vi "Exp05_JointAngle.vi"() -> ()   [LabVIEW 2019]
uses:
  <vilib>/myRIO/Instrument Drivers/Onboard IO/I2C/typedefs/I2C User Configuration.ctl
  <vilib>/myRIO/Instrument Drivers/Onboard IO/I2C/typedefs/I2C Transfer Rate.ctl
  <vilib>/Platform/TimedLoop/XDataNode/timing_clust.ctl
  <vilib>/Platform/TimedLoop/XDataNode/nitl_modes.ctl
  <vilib>/Platform/TimedLoop/XDataNode/wakeup.ctl
  <vilib>/Utility/error.llb/Error Cluster From Error Code.vi
  <vilib>/myRIO/Common/Instrument Driver Framework/myRIO v1.0/I2C/vis/myRIO v1.0 Configure I2C.vi
  <vilib>/myRIO/Common/Instrument Driver Framework/myRIO v1.0/I2C/vis/myRIO v1.0 Write I2C.vi
  <vilib>/myRIO/Common/Instrument Driver Framework/myRIO v1.0/I2C/vis/myRIO v1.0 Read I2C.vi
  <vilib>/Platform/TimedLoop/XDataNode/XDataNode.xnode
  <vilib>/myRIO/Instrument Drivers/Onboard IO/I2C/I2C.lvlib
  <vilib>/Platform/TimedLoop/XDataNode/XDNodeRunTimeDep.lvlib
panel:
  out "Joint Angle":dbl
  out "B/Angle":dbl
  out "A/Angle":dbl
  out "B/Acc X":i16
  out "B/Acc Y":i16
  out "B/Gyro Z":i16
  out "B/acc angle":dbl
  out "B/angular velocity":dbl
  in  "B/gyro_nitial_bias":i16
  in  "zero":bool
  in  "A/gyro_nitial_bias":i16
  out "A/angular velocity":dbl
  out "A/acc angle":dbl
  out "A/Gyro Z":i16
  out "A/Acc Y":i16
  out "A/Acc X":i16
  in  "stop":bool
  out "error out":errorcluster
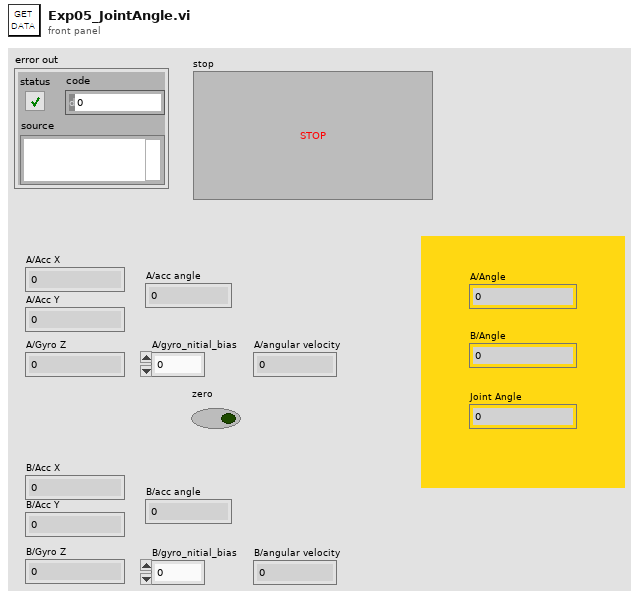
[diagram p1: front panel]
types:
  T1 = typedef "I2C.lvlib/I2C User Configuration.ctl" = cluster{"I2C Transfer Rate":T2}
  T2 = typedef "I2C.lvlib/I2C Transfer Rate.ctl" = enum16{"Standard mode (100 kbps)", "Fast mode (400 kbps)"}
  T3 = typedef "I2C.lvlib/I2C Reference.ctl" = cluster{"myRIO Reference":T4, "I2C Channels Enum":T8, "I2C Configuration":T9}
  T4 = typedef "myRIO Generic Hardware Reference.ctl" = cluster{"myRIO Model":T5, "myRIO Hardware Reference":T6}
  T5 = typedef "Hardware Version Enum.ctl" = enum16{"Unknown", "myRIO-1900", "myRIO-1950", "roboRIO", "NI ELVIS RIO CM", "ELVIS III"}
  T6 = typedef "myRIO v1.0 Reference.ctl" = cluster{"Generic FPGA Reference":T7, "Allow multiple opens":bool}
  T7 = typedef "Generic FPGA Reference.ctl" = refnum<k20>
  T8 = typedef "I2C Channels Enum.ctl" = enum16{"Not Connected", "A/I2C", "B/I2C", "I2C/I2C"}
  T9 = typedef "I2C.lvlib/I2C Configuration.ctl" = cluster{"I2C Transfer Rate":T2}
  T10 = typedef "XDNodeRunTimeDep.lvlib/timing_clust.ctl" = cluster{"Expected End [f-1]":u64, "Actual End [f-1]":u64, "Finished Late? [f-1]":bool, "Expected End [i-1]":u64, "Actual End [i-1]":u64, "Finished Late? [i-1]":bool, "Expected Start [i]":u64, "Actual Start [i]":u64, "Expected Start [f]":u64, "Actual Start [f]":u64, "Source Name":string, "Structure Name":string, "Period":i64, "Deadline":i64, "Offset":i64, "Start":i64, "Priority":i32, "Timeout":i32, "Mode":T11, "Wakeup Reason":T12, "Error":errorcluster, "Source Type":string, "Secondary Source Type":string, "Global End Time":u64, "Global Start Time":u64, "Frame Duration":u64, "Iteration Duration":u64, "Assigned CPU":i32, "I/O Scan Engine Mode":u32}
  T11 = typedef "XDNodeRunTimeDep.lvlib/nitl_modes.ctl" = enum32{"No Change", "Process missed periods, maintain original phase", "Discard missed periods, maintain original phase", "Process missed periods, ignore original phase", "Discard missed periods, ignore original phase"}
  T12 = typedef "XDNodeRunTimeDep.lvlib/wakeup.ctl" = enum32{"Normal", "Aborted", "Asynchronous wakeup", "Timing source error", "Timed loop error", "Timeout"}
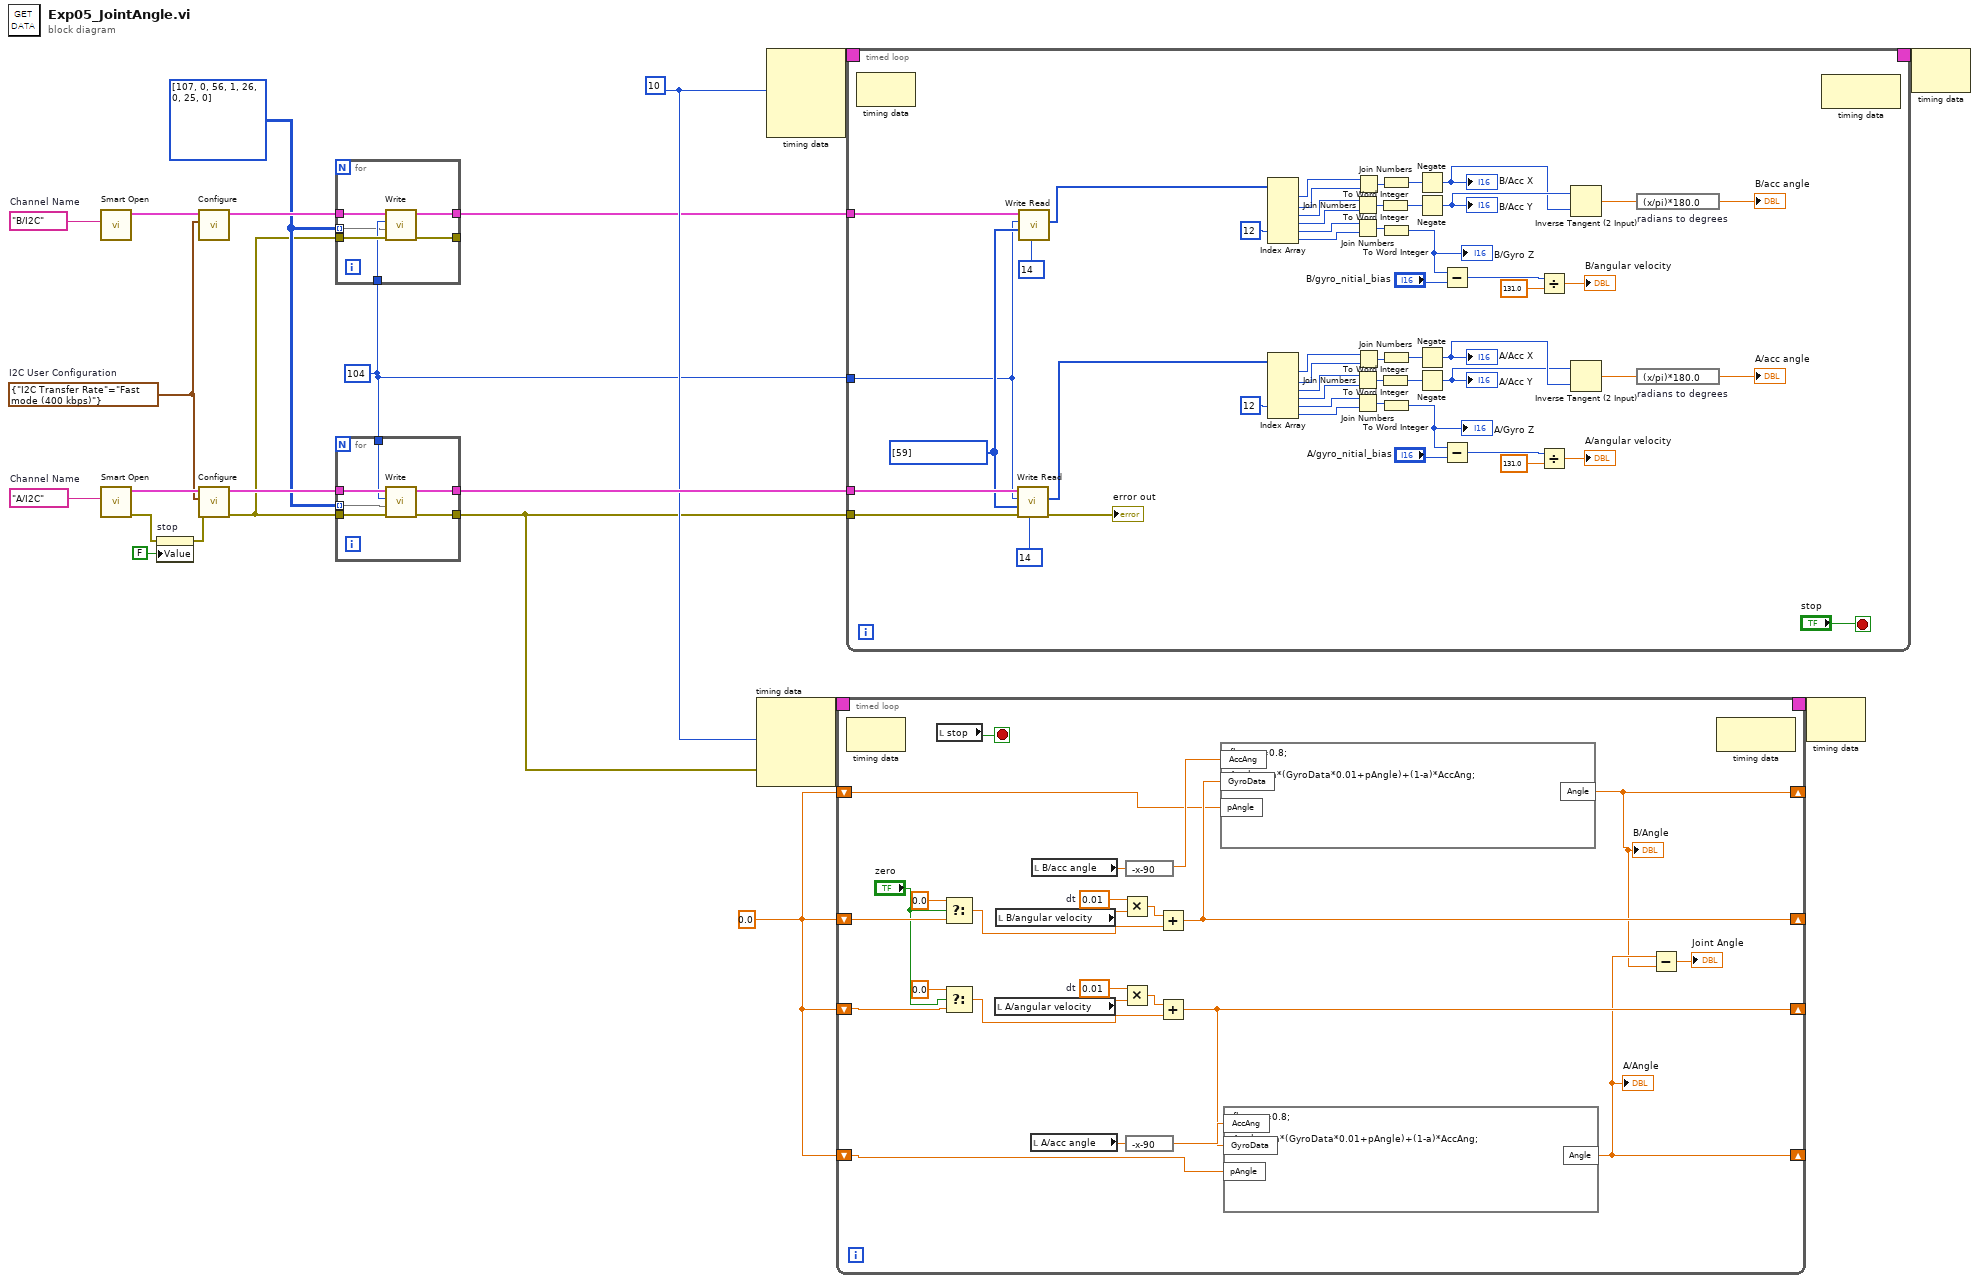
[diagram p0: block diagram]
diagram:
  w8 = tag "B/I2C"  # Channel Name
  w1 = 0.0
  w3 = u8 104 ("Slave Address (7-bit)")
  w11 = i64 10 ("Period")
  w5 = u8[][] [[107, 0], [56, 1], [26, 0], [25, 0]] ("Bytes to Write")
  w7 = T1 {"I2C Transfer Rate"=enum."Fast mode (400 kbps)"}  # I2C User Configuration
  w22 = tag "A/I2C"  # Channel Name
  n1 = call <vilib>:"Smart Open.vi"("Channel Name"=w8) -> ("I2C Ref Out"=w9:T3)  [unwired: 9 in, 1 out]
  n2 = call <vilib>:"Smart Open.vi"("Channel Name"=w22) -> ("error out"=w14:errorcluster, "I2C Ref Out"=w21:T3)  [unwired: 9 in]
  n3 = property on="stop" class="Bool (strict)"(error in=w14, "Value"=FALSE ("stop")) -> (error out=w12:errorcluster)  [unwired: 1 in, 1 out]
  n4 = call <vilib>:"Configure.vi"("I2C User Configuration"=w7, "I2C Ref In"=w9) -> ("I2C Ref Out"=w6:T3)  [unwired: 8 in, 1 out]
  n5 = call <vilib>:"Configure.vi"("error in (no error)"=w12, "I2C User Configuration"=w7, "I2C Ref In"=w21) -> ("error out"=w4:errorcluster, "I2C Ref Out"=w17:T3)  [unwired: 7 in]
  n6 = for {
    tunnel: w3 -> [w24]
    tunnel: w6 -> [w28]
    tunnel: [w25] -> w2
    tunnel: w4 -> [w27]
    tunnel: [w26] -> _
    tunnel: w5 -> [w23] mode=indexing
    n7 = call <vilib>:"Write.vi"("error in (no error)"=w27, "Bytes to Write"=w23, "Slave Address (7-bit)"=w24, "I2C Ref In"=w28) -> ("error out"=w26:errorcluster, "I2C Ref Out"=w25:T3)  [unwired: 6 in]
  }
  n8 = for {
    tunnel: w3 -> [w30]
    tunnel: w17 -> [w34]
    tunnel: [w31] -> w20
    tunnel: w4 -> [w33]
    tunnel: [w32] -> w10
    tunnel: w5 -> [w29] mode=indexing
    n9 = call <vilib>:"Write.vi"("error in (no error)"=w33, "Bytes to Write"=w29, "Slave Address (7-bit)"=w30, "I2C Ref In"=w34) -> ("error out"=w32:errorcluster, "I2C Ref Out"=w31:T3)  [unwired: 6 in]
  }
  n10 = node-c288(w11, w10) -> (w16:T10)  [unwired: 2 in]
  n11 = node-c288(w11) -> (w19:T10)  [unwired: 3 in]
  n12 = timed-loop {
    timing: w16 -> [_]
    timing-out: [_] -> w15
    shift-right: [w50] -> _
    shift-left: w1 -> [w55]
    shift-right: [w36] -> _
    shift-left: w1 -> [w49]
    shift-right: [w37] -> _
    shift-left: w1 -> [w40]
    shift-right: [w39] -> _
    shift-left: w1 -> [w38]
    stop <- w53 stop-if-true
    w44 = 0.01  # dt
    w58 = 0.01  # dt
    n13 = node-c288() -> ()  [unwired: 1 in, 1 out]
    n14 = local read "stop"() -> (w53:bool)
    n15 = Select(t=0.0, s="zero", f=w55) -> (s? t:f=w54:dbl)
    n16 = Select(t=0.0, s="zero", f=w38) -> (s? t:f=w47:dbl)
    n17 = local read "A/angular velocity"() -> (w43:dbl)
    n18 = local read "B/angular velocity"() -> (w59:dbl)
    n19 = local read "A/acc angle"() -> (w48:dbl)
    n20 = local read "B/acc angle"() -> (w52:dbl)
    n21 = Multiply(x=w58, y=w59) -> (x*y=w57:dbl)
    n22 = Multiply(x=w44, y=w43) -> (x*y=w45:dbl)
    n23 = expression code="-x-90"(w52) -> (w51:dbl)
    n24 = expression code="-x-90"(w48) -> (w42:dbl)
    n25 = Add(x=w57, y=w54) -> (x+y=w50:dbl)
    n26 = Add(x=w45, y=w47) -> (x+y=w39:dbl)
    n27 = formula code="float a=0.8;\n\nAngle = a*(GyroData*0.01+pAngle)+(1-a)*AccAng;"("AccAng"=w51, "GyroData"=w50, "pAngle"=w49) -> ("Angle"=w36:dbl)
    "B/Angle" <- w36
    n28 = formula code="float a=0.8;\n\nAngle = a*(GyroData*0.01+pAngle)+(1-a)*AccAng;"("AccAng"=w42, "GyroData"=w39, "pAngle"=w40) -> ("Angle"=w37:dbl)
    "A/Angle" <- w37
    n29 = Subtract(x=w37, y=w36) -> (x-y=→"Joint Angle":dbl)
    n30 = node-c288() -> ()  [unwired: 1 in, 1 out]
  }
  n31 = timed-loop {
    timing: w19 -> [_]
    timing-out: [_] -> w18
    tunnel: w10 -> [w112]
    tunnel: w20 -> [w111]
    tunnel: w3 -> [w87]
    tunnel: w2 -> [w89]
    stop <- "stop" stop-if-true
    w88 = u8[] [59] ("Bytes to Write")
    n32 = node-c288() -> ()  [unwired: 1 in, 1 out]
    n33 = call <vilib>:"Write Read.vi"("Byte Count"=u32 14, "error in (no error)"=w112, "Bytes to Write"=w88, "Slave Address (7-bit)"=w87, "I2C Ref In"=w111) -> ("error out"=→"error out":errorcluster, "Bytes Read"=w100:u8[])  [unwired: 3 in, 1 out]
    n34 = call <vilib>:"Write Read.vi"("Byte Count"=u32 14, "Bytes to Write"=w88, "Slave Address (7-bit)"=w87, "I2C Ref In"=w89) -> ("Bytes Read"=w62:u8[])  [unwired: 4 in, 2 out]
    n35 = Index Array(array=w62, index #5=12 ("index")) -> (element #1=w63:u8, element #2=w64:u8, element #3=w65:u8, element #4=w66:u8, element #5=w67:u8, element #6=w68:u8)  [unwired: 5 in]
    n36 = Index Array(array=w100, index #5=12 ("index")) -> (element #1=w109:u8, element #2=w108:u8, element #3=w107:u8, element #4=w106:u8, element #5=w105:u8, element #6=w104:u8)  [unwired: 5 in]
    n37 = Join Numbers(hi=w65, lo=w66) -> ((hi.lo)=w70:u16)
    n38 = Join Numbers(hi=w67, lo=w68) -> ((hi.lo)=w71:u16)
    n39 = Join Numbers(hi=w107, lo=w106) -> ((hi.lo)=w102:u16)
    n40 = Join Numbers(hi=w105, lo=w104) -> ((hi.lo)=w101:u16)
    n41 = Join Numbers(hi=w63, lo=w64) -> ((hi.lo)=w69:u16)
    n42 = Join Numbers(hi=w109, lo=w108) -> ((hi.lo)=w103:u16)
    n43 = To Word Integer(number=w70) -> (16bit integer=w76:i16)
    n44 = To Word Integer(number=w102) -> (16bit integer=w95:i16)
    n45 = To Word Integer(number=w69) -> (16bit integer=w74:i16)
    n46 = To Word Integer(number=w71) -> (16bit integer=w82:i16)
    "B/Gyro Z" <- w82
    n47 = To Word Integer(number=w103) -> (16bit integer=w97:i16)
    n48 = To Word Integer(number=w101) -> (16bit integer=w85:i16)
    "A/Gyro Z" <- w85
    n49 = Negate(x=w74) -> (-x=w75:i16)
    "B/Acc X" <- w75
    n50 = Negate(x=w76) -> (-x=w77:i16)
    "B/Acc Y" <- w77
    n51 = Negate(x=w97) -> (-x=w96:i16)
    "A/Acc X" <- w96
    n52 = Negate(x=w95) -> (-x=w94:i16)
    "A/Acc Y" <- w94
    n53 = Subtract(x=w82, y="B/gyro_nitial_bias") -> (x-y=w81:i16)
    n54 = Subtract(x=w85, y="A/gyro_nitial_bias") -> (x-y=w90:i16)
    n55 = Divide(x=w81, y=131.0) -> (x/y=→"B/angular velocity":dbl)
    n56 = Divide(x=w90, y=131.0) -> (x/y=→"A/angular velocity":dbl)
    n57 = Inverse Tangent (2 Input)(1:w75, 2:w77) -> (0:w72:dbl)
    n58 = Inverse Tangent (2 Input)(1:w96, 2:w94) -> (0:w99:dbl)
    n59 = expression code="(x/pi)*180.0" "radians to degrees"(w72) -> (→"B/acc angle":dbl)
    n60 = expression code="(x/pi)*180.0" "radians to degrees"(w99) -> (→"A/acc angle":dbl)
    n61 = node-c288() -> ()  [unwired: 1 in, 1 out]
  }
  n62 = node-c288(w15) -> ()  [unwired: 1 out]
  n63 = node-c288(w18) -> ()  [unwired: 1 out]
